vi "Data File Processing UI Variable.vi"() -> (8 "Virance":cluster{"error":errorcluster})   [LabVIEW 2011]
panel:
  in  "error":errorcluster
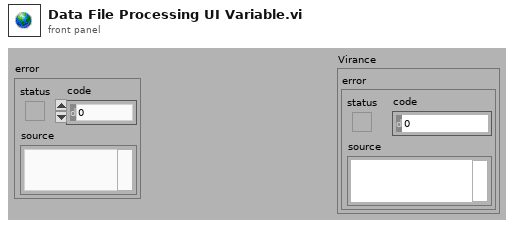
[diagram p1: front panel]
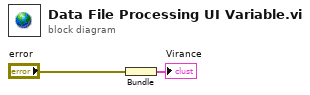
[diagram p0: block diagram]
diagram:
  n1 = Bundle("error"="error") -> (→"Virance":cluster{"error":errorcluster})  [unwired: 1 in]
